vi "Data Save.vi"(6 "Test Type":u8[](array[numeric]), 7 "Test Trial In Progress":string, 8 "Error IN":errorcluster, 9 "Trial#":i16, 10 "Data Cluster":T1 {"Seconds Into Trial(s)" format="%#.10g"}, 11 "Task":T2(ring)) -> (0 "Error OUT":errorcluster, 3 "Data Save Path":path)   [LabVIEW 2018]
uses:
  controls/Data To Save.ctl
  <vilib>/Utility/file.llb/Write Delimited Spreadsheet (string).vi
panel:
  out "T2":path
  out "T1":path
  out "Save Directory OUT":path
  out "\"Create Folder\", Default":errorcluster
  out "\"Create Folder\", Default":path
  out "error out 2":errorcluster
  out "error out":errorcluster
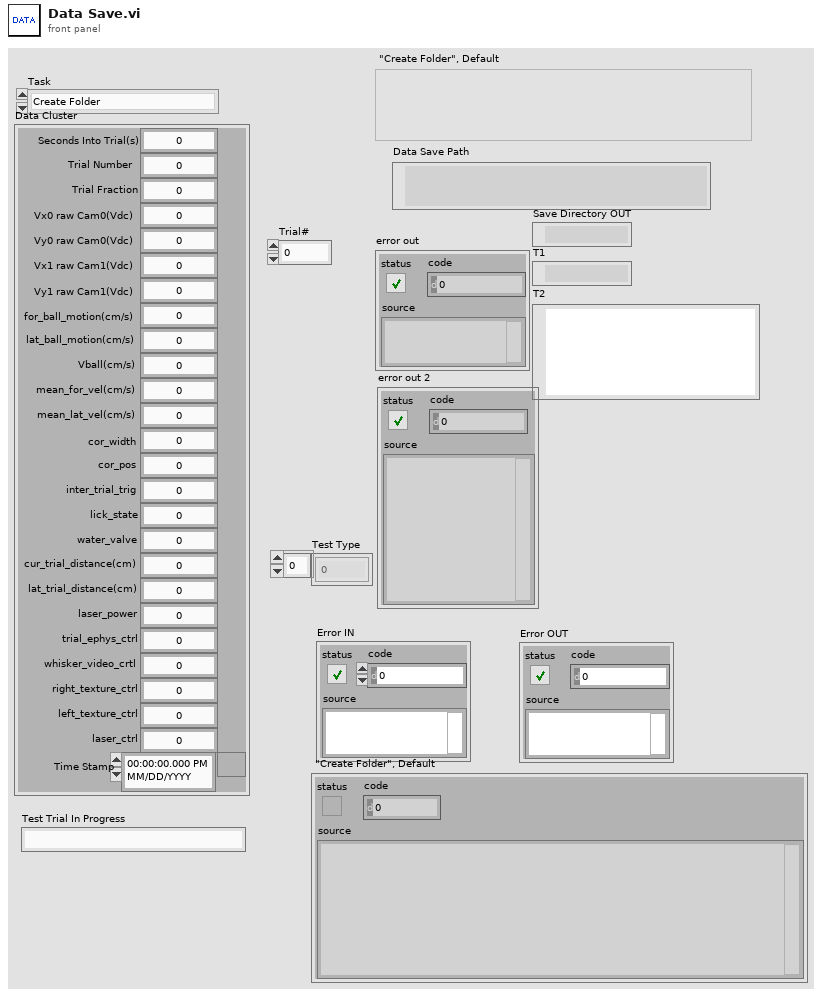
[diagram p1: front panel]
types:
  T1 = typedef "Data To Save.ctl" = cluster{"Vx0 raw Cam0(Vdc)":sgl, "Vy0 raw Cam0(Vdc)":sgl, "Vx1 raw Cam1(Vdc)":sgl, "Vy1 raw Cam1(Vdc)":sgl, "Seconds Into Trial(s)":dbl, "cor_width":sgl, "cor_pos":sgl, "for_ball_motion(cm/s)":sgl, "lat_ball_motion(cm/s)":sgl, "Vball(cm/s)":sgl, "mean_for_vel(cm/s)":sgl, "mean_lat_vel(cm/s)":sgl, "Trial Fraction":dbl, "Trial Number":i16, "inter_trial_trig":i16, "lick_state":i16, "water_valve":i16, "cur_trial_distance(cm)":dbl, "lat_trial_distance(cm)":dbl, "laser_power":dbl, "trial_ephys_ctrl":i16, "whisker_video_crtl":i16, "right_texture_ctrl":i16, "left_texture_ctrl":i16, "laser_ctrl":i16, "Time Stamp":timestamp}
  T2 = enum16{"Create Folder", "Save", "Create New Data File"}
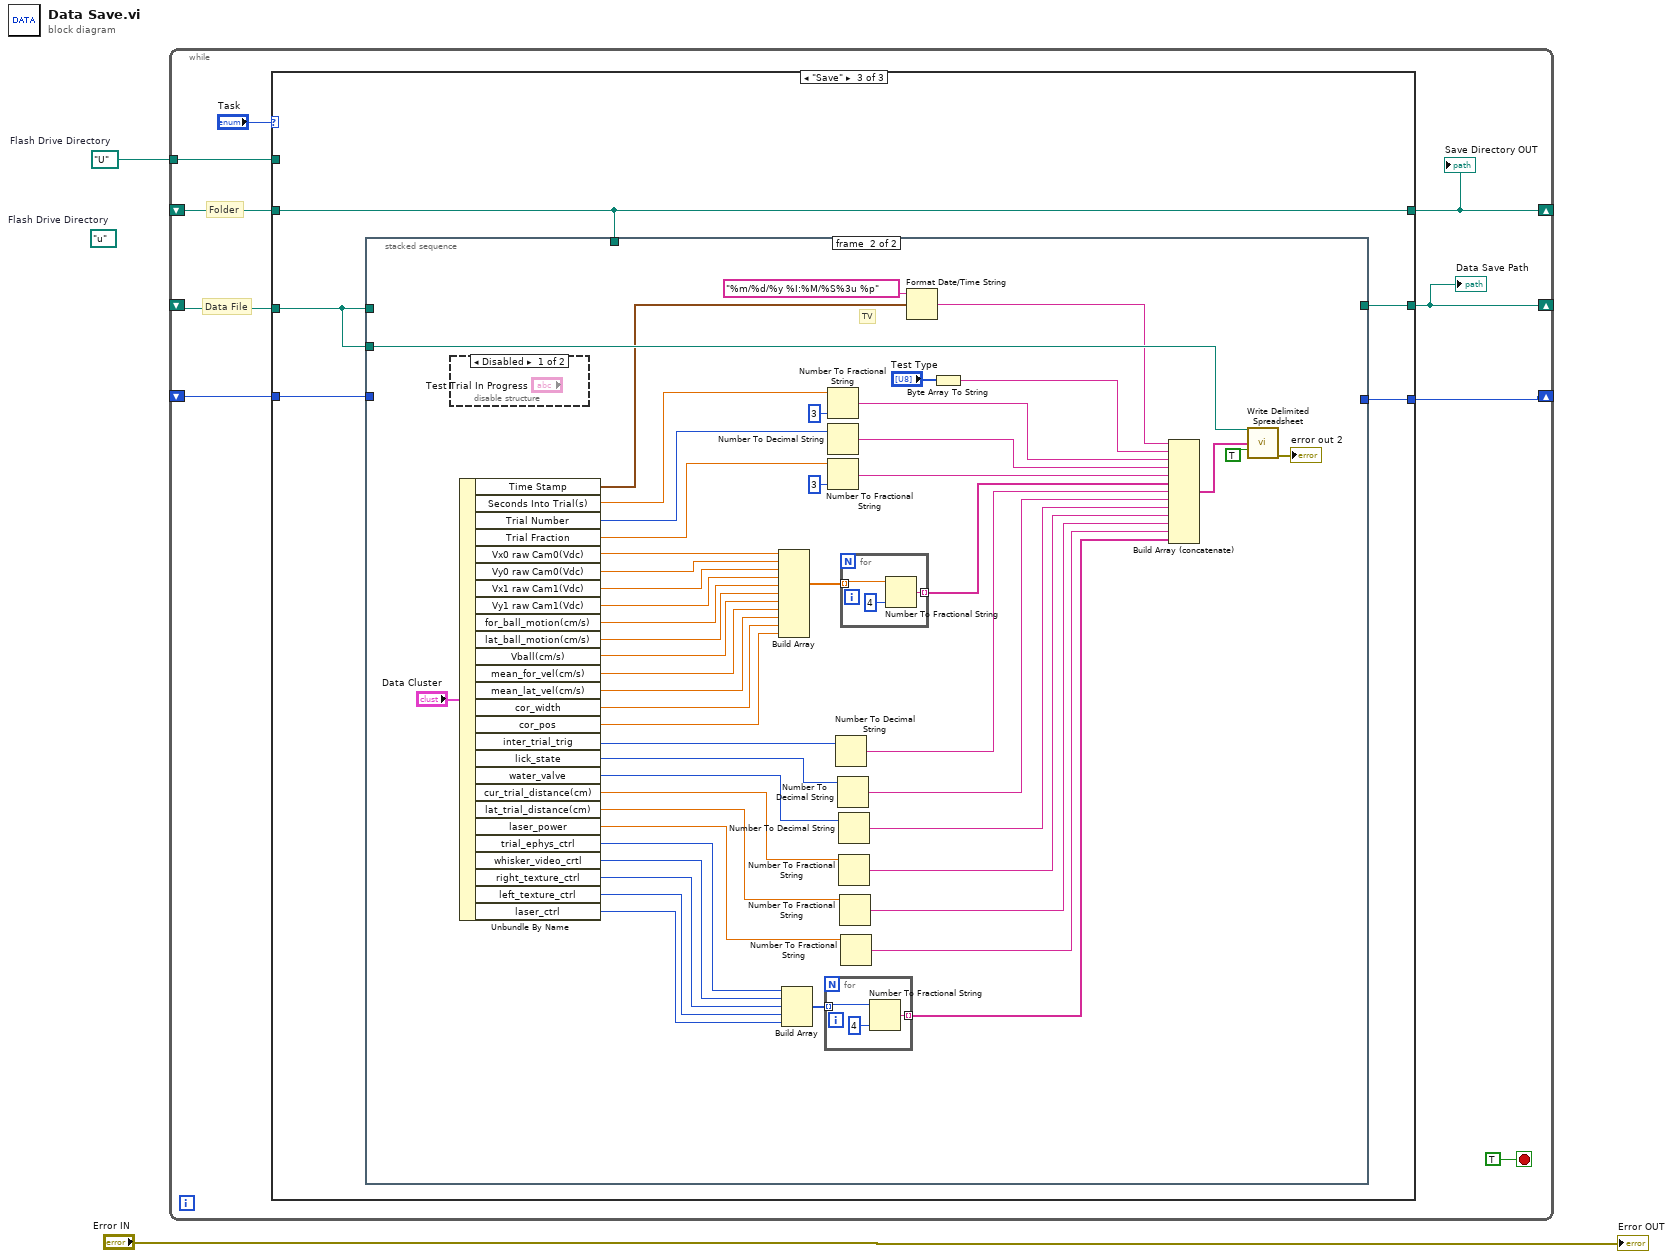
[diagram p0: block diagram]
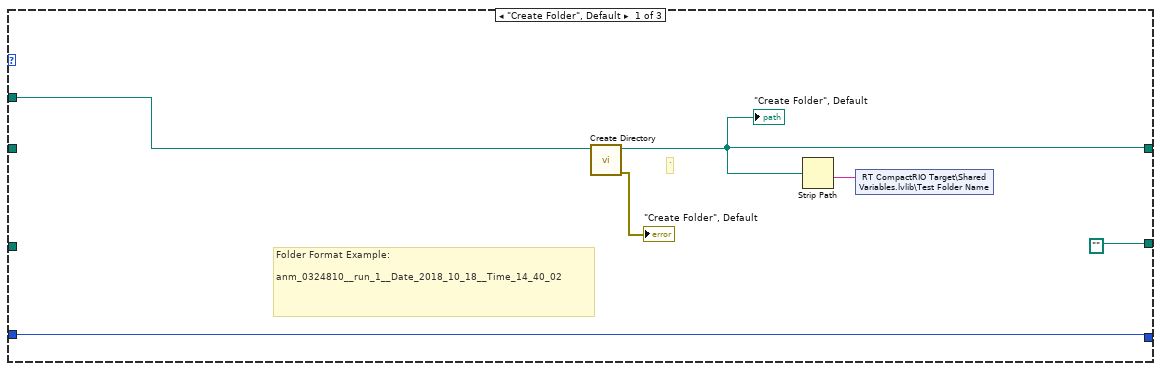
[diagram p2: hidden frame]
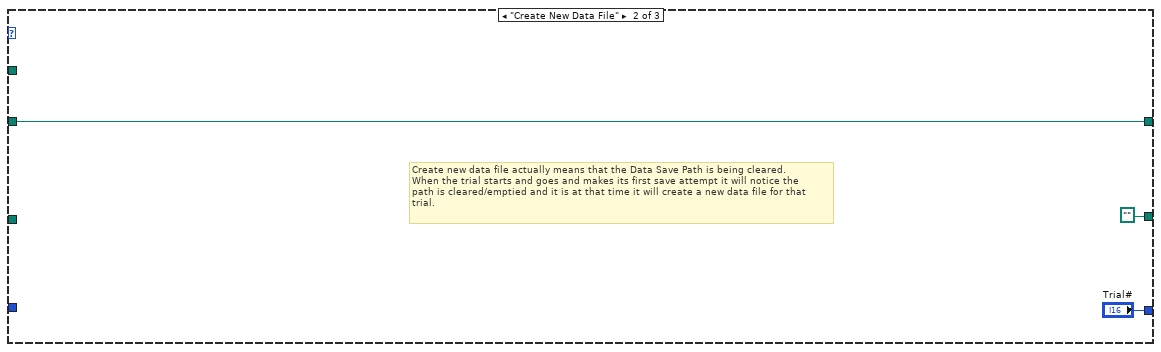
[diagram p3: hidden frame]
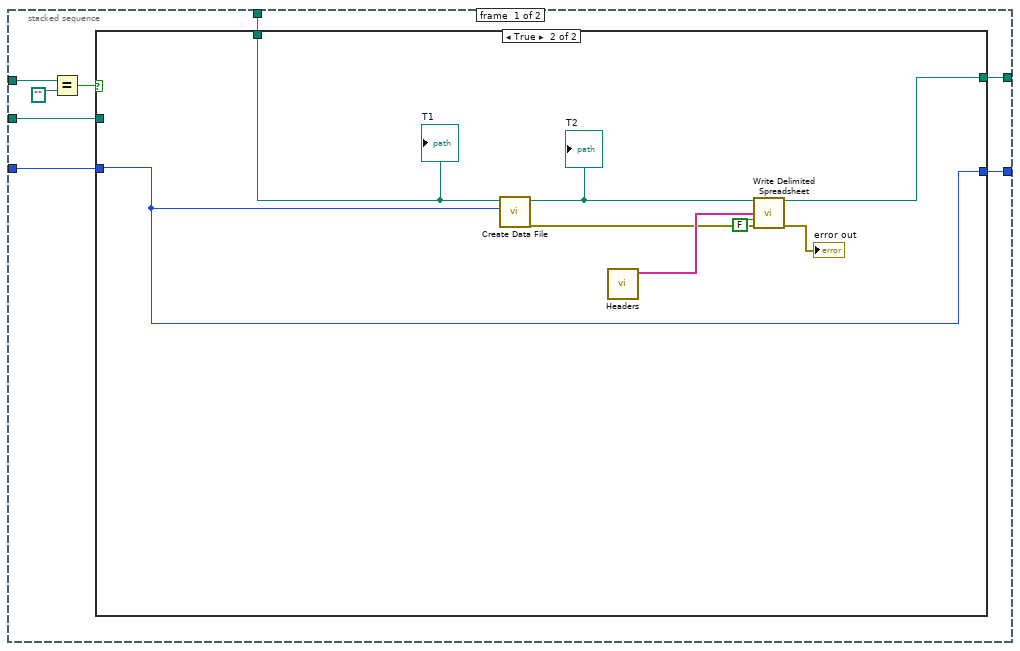
[diagram p4: hidden frame]
diagram:
  (unwired) path "u:/"  # Flash Drive Directory
  w2 = path "U:/"  # Flash Drive Directory
  n1 = while {
    shift-right: [w8] -> _
    shift-left: _ -> [w9]
    tunnel: w2 -> [w7]
    shift-right: [w5] -> _
    shift-left: _ -> [w6]
    shift-right: [w4] -> _
    shift-left: _ -> [w3]
    stop <- TRUE stop-if-true
    # "Data File"
    # "Folder"
    n2 = case shown="\"Save\"" "Task" {
      tunnel: w9 -> [_ w19 w25]
      tunnel: [w14 w19 w25] -> w8
      tunnel: w7 -> [w17 _ _]
      tunnel: [path "" path "" w24] -> w5
      tunnel: w6 -> [_ _ w23]
      tunnel: [w12 "Trial#" w21] -> w4
      tunnel: w3 -> [w12 _ w22]
      frame "Create Folder", Default {
        # "`"
        # "Folder Format Example:\n\nanm_0324810__run_1__Date_2018_10_18__Time_14_40_02"
        n3 = call "Create Directory.vi"("Default Save Directory IN"=w17) -> ("Error OUT"=→"\"Create Folder\", Default":errorcluster, "Save Directory OUT"=w14:path)  [unwired: 9 in]
        "\"Create Folder\", Default" <- w14
        n4 = Strip Path(path=w14) -> (name=w13:string)  [unwired: 1 out]
        n5 = shared-variable "RT CompactRIO Target\\Shared Variables.lvlib\\Test Folder Name"(w13) -> ()  [unwired: 1 in, 1 out]
      }
      frame "Create New Data File" {
        # "Create new data file actually means that the Data Save Path is being cleared.\nWhen the trial starts and goes and makes its first save attempt it will notice the\npath is cleared/emptied and it is at that time it will create a new data file for that\ntrial."
      }
      frame "Save" {
        n6 = stacked-sequence {
          tunnel: w23 -> [w33 _]
          tunnel: w25 -> [w30 _]
          tunnel: [w29 _] -> w24
          tunnel: w23 -> [w28 w93]
          tunnel: w22 -> [w27 _]
          tunnel: [w26 _] -> w21
          frame #0 {
            n7 = Equal?(x=w33, y=path "") -> (x = y?=w31:bool)
            n8 = case shown="True" w31 {
              tunnel: w30 -> [_ w41]
              tunnel: [w35 w39] -> w29
              tunnel: w28 -> [w35 _]
              tunnel: w27 -> [w34 w36]
              tunnel: [w34 w36] -> w26
              frame False {
              }
              frame True {
                n9 = call "Create Data File.vi"("Trial#"=w36, "Save Directory IN"=w41) -> ("Error OUT"=w38:errorcluster, "Data File Path OUT"=w40:path)  [unwired: 8 in]
                "T2" <- w40
                n10 = call "Headers.vi"() -> ("Header Array OUT"=w43:string[])  [unwired: 11 in]
                n11 = call-poly <vilib>:"Write Delimited Spreadsheet.vi"("file path (dialog if empty)"=w40, "1D data"=w43, "append to file? (new file:F)"=FALSE, "error in (no error)"=w38) -> ("new file path (Not A Path if cancelled)"=w39:path, "error out"=→"error out":errorcluster)  [unwired: 10 in]
                "T1" <- w41
              }
            }
          }
          frame #1 {
            # "TV"
            n12 = disable-structure shown="Disabled" {
              frame Disabled {
              }
              frame Enabled {
              }
            }
            n13 = Unbundle By Name("Data Cluster") -> ("Time Stamp"=w47:timestamp, "Seconds Into Trial(s)"=w78:dbl, "Trial Number"=w76:i16, "Trial Fraction"=w49:dbl, "Vx0 raw Cam0(Vdc)"=w89:sgl, "Vy0 raw Cam0(Vdc)"=w88:sgl, "Vx1 raw Cam1(Vdc)"=w87:sgl, "Vy1 raw Cam1(Vdc)"=w86:sgl, "for_ball_motion(cm/s)"=w85:sgl, "lat_ball_motion(cm/s)"=w84:sgl, "Vball(cm/s)"=w83:sgl, "mean_for_vel(cm/s)"=w82:sgl, "mean_lat_vel(cm/s)"=w81:sgl, "cor_width"=w71:sgl, "cor_pos"=w70:sgl, "inter_trial_trig"=w69:i16, "lick_state"=w68:i16, "water_valve"=w65:i16, "cur_trial_distance(cm)"=w63:dbl, "lat_trial_distance(cm)"=w50:dbl, "laser_power"=w60:dbl, "trial_ephys_ctrl"=w58:i16, "whisker_video_crtl"=w57:i16, "right_texture_ctrl"=w56:i16, "left_texture_ctrl"=w55:i16, "laser_ctrl"=w54:i16)
            n14 = Build Array(w89, w88, w87, w86, w85, w84, w83, w82, w81, w71, w70) -> (w80:sgl[])
            n15 = Build Array(w58, w57, w56, w55, w54) -> (w53:i16[])
            n16 = for {
              tunnel: w53 -> [w95] mode=indexing
              tunnel: [w94] -> w52 mode=indexing
              n17 = Number To Fractional String(number=w95, precision (6)=i16 4) -> (F-format string=w94:string)  [unwired: 2 in]
            }
            n18 = Number To Fractional String(number=w78, precision (6)=i16 3) -> (F-format string=w77:string)  [unwired: 2 in]
            n19 = Number To Decimal String(number=w76) -> (decimal integer string=w75:string)  [unwired: 1 in]
            n20 = Number To Fractional String(number=w49, precision (6)=i16 3) -> (F-format string=w73:string)  [unwired: 2 in]
            n21 = Number To Decimal String(number=w69) -> (decimal integer string=w67:string)  [unwired: 1 in]
            n22 = Number To Decimal String(number=w68) -> (decimal integer string=w66:string)  [unwired: 1 in]
            n23 = Number To Decimal String(number=w65) -> (decimal integer string=w64:string)  [unwired: 1 in]
            n24 = Number To Fractional String(number=w63) -> (F-format string=w62:string)  [unwired: 3 in]
            n25 = Number To Fractional String(number=w50) -> (F-format string=w61:string)  [unwired: 3 in]
            n26 = for {
              tunnel: w80 -> [w98] mode=indexing
              tunnel: [w97] -> w72 mode=indexing
              n27 = Number To Fractional String(number=w98, precision (6)=i16 4) -> (F-format string=w97:string)  [unwired: 2 in]
            }
            n28 = Number To Fractional String(number=w60) -> (F-format string=w59:string)  [unwired: 3 in]
            n29 = Format Date/Time String(time format string (%c)="%m/%d/%y %I:%M/%S%3u %p", seconds (now)=w47) -> (date/time string=w46:string)  [unwired: 1 in]
            n30 = Byte Array To String(unsigned byte array="Test Type") -> (string=w44:string)
            n31 = Build Array (concatenate)(w46, w44, w77, w75, w73, w72, w67, w66, w64, w62, w61, w59, w52) -> (w92:string[])
            n32 = call-poly <vilib>:"Write Delimited Spreadsheet.vi"("file path (dialog if empty)"=w93, "1D data"=w92, "append to file? (new file:F)"=TRUE) -> ("error out"=→"error out 2":errorcluster)  [unwired: 11 in, 1 out]
          }
        }
      }
    }
    "Data Save Path" <- w5
    "Save Directory OUT" <- w8
  }
  "Error OUT" <- "Error IN"
